vi "ROI entry-Clear image.vi"(8 "error in (no error)":errorcluster) -> (0 "error out":errorcluster)   [LabVIEW 2020]
uses:
  ROI Entry screen/Globals/gl_ROI Entry UI globals.vi
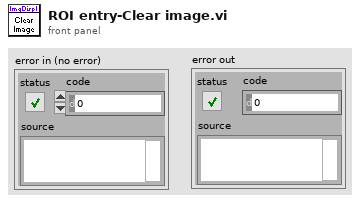
[diagram p1: front panel]
types:
  T1 = typedef "ROI entry screen ctrl refs cluster.ctl" = cluster{"Done button":refnum<vi>, "Imaging button":refnum<vi>, "Acquisition button":refnum<vi>, "Scan dwell time per pixel (us)":refnum<vi>, "# of planes":refnum<vi>, "Zoom Ctrl":refnum<vi>, "Equal size":refnum<vi>, "Channel":refnum<vi>, "Image Display":refnum<vi>, "Z-Plane Selector":refnum<vi>, "Number of lines left":refnum<vi>, "Z-stack folder path":refnum<vi>, "POI Density":refnum<vi>, "Arb Plane Entry":refnum<vi>, "Whole Plane":refnum<vi>, "Line Mode":refnum<vi>, "Clear Last":refnum<vi>, "Clear All":refnum<vi>, "Delete Lines":refnum<vi>, "Trial Length (sec)":refnum<vi>, "Palette Type":refnum<vi>, "Intensity slider":refnum<vi>, "# POI":refnum<vi>, "Max Z Proj":refnum<vi>, "Zplane ind":refnum<vi>, "Wavelength (nm)":refnum<vi>, "Number of Trials":refnum<vi>, "Funct stim.trig.enable":refnum<vi>, "Funct stim.trig.delay (s)":refnum<vi>, "Line Mode":refnum<vi>, "Step size (µm)":refnum<vi>, "ROI move mode":refnum<vi>, "Cool-down time (s)":refnum<vi>, "Enable cool-down time":refnum<vi>, "Motor Z ind. (um)":refnum<vi>, "AOL Z ind. (um)":refnum<vi>, "Load Reference Image":refnum<vi>, "Rel.  Res.":refnum<vi>, "ROI LIST":refnum<vi>, "Show All":refnum<vi>, "ROI Type":refnum<vi>, "Start Plane":refnum<vi>, "Stop Plane":refnum<vi>, "Offset ROI":refnum<vi>, "Tab Control":refnum<vi>, "Laser Power(%)":refnum<vi>, "Cycle rate":refnum<vi>, "FOV (Ind.)":refnum<vi>, "Frame Size (Ind.)":refnum<vi>, "Resolution (Ind.)":refnum<vi>, "Pixel Density (Ind)":refnum<vi>, "Laser Power (Ind.)":refnum<vi>, "Dwell Time (Ind.)":refnum<vi>, "Adj MC":refnum<vi>}
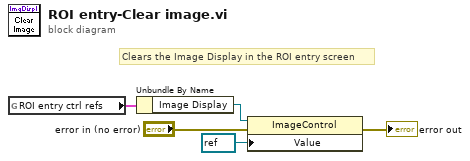
[diagram p0: block diagram]
diagram:
  # "Clears the Image Display in the ROI entry screen"
  n1 = global read "gl_ROI Entry UI globals.vi" "ROI entry ctrl refs"() -> (w5:T1)
  n2 = Unbundle By Name(w5) -> ("Image Display"=w3:refnum<vi>)
  n3 = property on="Property Node" class="ImageControl"(reference=w3, error in="error in (no error)", "Value"=refnum<image> refnum ("Zstack")) -> (error out=→"error out":errorcluster)  [unwired: 1 out]
